vi "Type Conversion.From Double.Subset (1D I16).vi"(9 "index (0)":i64, 10 "count":i64, 11 "values in":dbl[](array[numeric])) -> (2 "converted values out":i16[](array[numeric]), 3 "values out":dbl[](array[numeric]))   [LabVIEW 2016, in "VeriStand Data.lvlib"]
doc: "Converts the provided double float values to the specified data type, preserving the numerical value of the data."
uses:
  VeriStand Data.lvlib
  Type Conversion.From Double (1D I16).vi
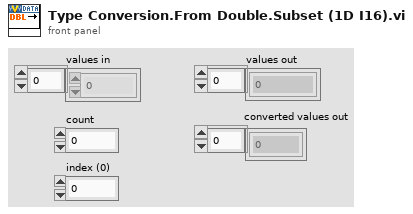
[diagram p1: front panel]
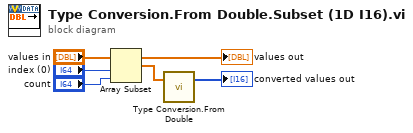
[diagram p0: block diagram]
diagram:
  n1 = Array Subset(array="values in", index="index (0)", length="count") -> (w2:dbl[])
  n2 = call-poly "Type Conversion.From Double.vi"("values in"=w2) -> ("values out"=→"converted values out":i16[])  [unwired: 2 in]
  "values out" <- "values in"
